vi "MotPrg.vi"() -> ()   [LabVIEW 2013]
panel:
  out "Chaîne":string
  in  "Fonctions":enum16{"Voltmètre", "Amperemetre", "Ohmmetre"}(ring)
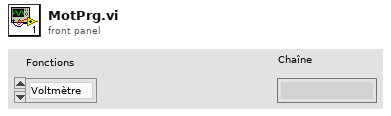
[diagram p1: front panel]
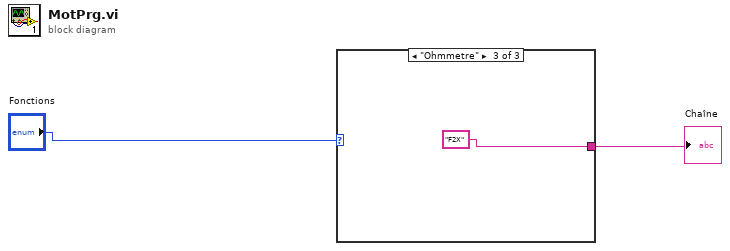
[diagram p0: block diagram]
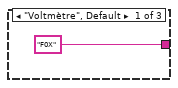
[diagram p2: hidden frame]
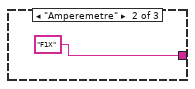
[diagram p3: hidden frame]
diagram:
  n1 = case shown="\"Ohmmetre\"" "Fonctions" {
    tunnel: ["F0X" "F1X" "F2X"] -> w1
    frame "Voltmètre", Default {
    }
    frame "Amperemetre" {
    }
    frame "Ohmmetre" {
    }
  }
  "Chaîne" <- w1
